vi "Calculate Transition Length.vi"(8 "error in (no error)":errorcluster, 9 "30-70 Rise":dbl, 10 "1/ fSCL":dbl, 11 "I2C timing (ticks)":T1) -> (0 "error out":errorcluster, 3 "I2C timing (ticks) out":T1)   [LabVIEW 2009, in "IDW.lvlib"]
doc: "Computes the length of the undefined transition region where no particular data is required to exist."
uses:
  IDW.lvlib
  _Typedefs/Timing - ticks.ctl
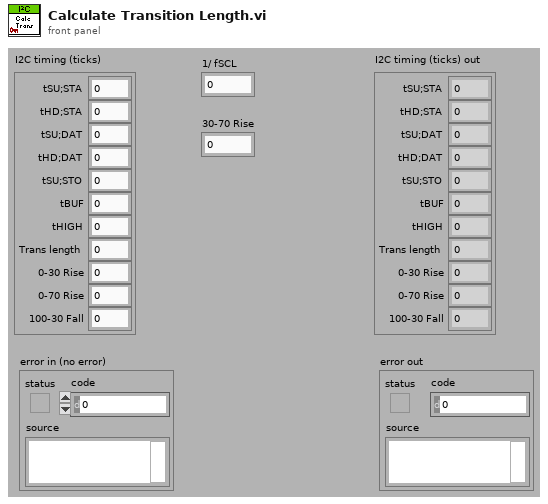
[diagram p1: front panel]
types:
  T1 = typedef "IDW.lvlib/Timing - ticks.ctl" = cluster{"tSU;STA":i32, "tHD;STA":i32, "tSU;DAT":i32, "tHD;DAT":i32, "tSU;STO":i32, "tBUF":i32, "tHIGH":i32, "Trans length":i32, "0-30 Rise":i32, "0-70 Rise":i32, "100-30 Fall":i32}
  T2 = cluster{"tSU;STA":dbl, "tHD;STA":dbl, "tSU;DAT":dbl, "tHD;DAT":dbl, "tSU;STO":dbl, "tBUF":dbl, "tHIGH":dbl, "Trans length":dbl, "0-30 Rise":dbl, "0-70 Rise":dbl, "100-30 Fall":dbl}
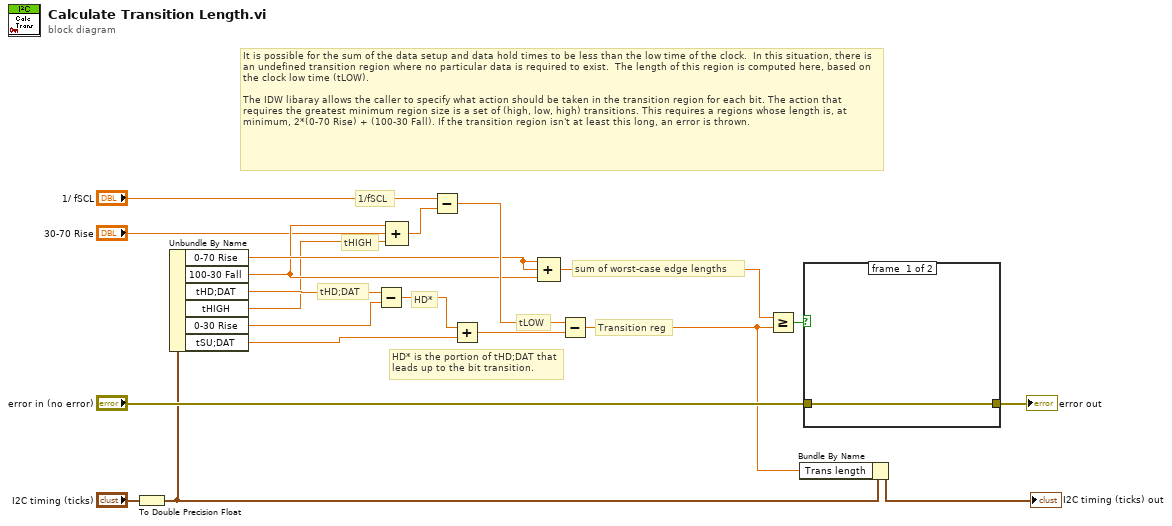
[diagram p0: block diagram]
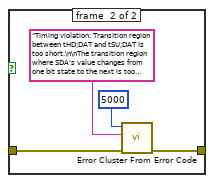
[diagram p2: hidden frame]
diagram:
  # "HD* is the portion of tHD;DAT that leads up to the bit transition."
  # "sum of worst-case edge lengths"
  # "1/fSCL"
  # "Transition reg"
  # "HD*"
  # "tHD;DAT"
  # "tHIGH"
  # "It is possible for the sum of the data setup and data hold times to be less than the low time of the clock.  In this situation, there is an undefined transition region where no particular data is required to exist.  The length of this region is computed here, based on the clock low time (tLOW).\n\nThe IDW libaray allows the caller to specify what action should be taken in the transition region for each bit. The action that requires the greatest minimum region size is a set of (high, low, high) transitions. This requires a regions whose length is, at minimum, 2*(0-70 Rise) + (100-30 Fall). If the transition region isn't at least this long, an error is thrown."
  # "tLOW"
  n1 = To Double Precision Float(number="I2C timing (ticks)") -> (double precision float=w9:T2)
  n2 = Unbundle By Name(w9) -> ("0-70 Rise"=w6:dbl, "100-30 Fall"=w5:dbl, "tHD;DAT"=w20:dbl, "tHIGH"=w2:dbl, "0-30 Rise"=w3:dbl, "tSU;DAT"=w19:dbl)
  n3 = Subtract(x=w20, y=w3) -> (x-y=w13:dbl)
  n4 = Compound Arithmetic op=ADD(w5, "30-70 Rise", w2) -> (w14:dbl)
  n5 = Subtract(x="1/ fSCL", y=w14) -> (x-y=w15:dbl)
  n6 = Add(x=w13, y=w19) -> (x+y=w16:dbl)
  n7 = Compound Arithmetic op=ADD(w6, w6, w5) -> (w18:dbl)
  n8 = Subtract(x=w15, y=w16) -> (x-y=w8:dbl)
  n9 = Greater Or Equal?(x=w18, y=w8) -> (x >= y?=w17:bool)
  n10 = Bundle By Name(cluster=w9, "Trans length"=w8) -> (→"I2C timing (ticks) out":T2)
  n11 = case shown="True" w17 {
    tunnel: [w21 w24] -> w11
    tunnel: "error in (no error)" -> [w21 w25]
    frame #0 {
    }
    frame #1 {
      n12 = call <vilib>:"Error Cluster From Error Code.vi"("error in (no error)"=w25, "error message (\"\")"="Timing violation: Transition region between tHD;DAT and tSU;DAT is too short.\n\nThe transition region where SDA's value changes from one bit state to the next is too short. This region's length is roughly equal to tLOW - (tHD;DAT + tSU;DAT). Its length must be no less than 2*(0-70 Rise) + (100-30 Fall) in order to accommodate all possible transition actions.\n\nYou must do one or more of the following:\n- Increase tLOW by decreasing fSCL or increasing tHIGH)\n- Decrease tHD;DAT\n- Decrease tSU;DAT\n\nYou may also choose to disregard the rise and fall times of edges by setting all parameters in the \"I/O timing (ns)\" cluster to 0." ("error message (\"\")"), "error code (0)"=5000) -> ("error out"=w24:errorcluster)  [unwired: 1 in, 5 out]
    }
  }
  "error out" <- w11
